vi "oa_Init N Channel Analog Tacho Process Paramters.vi"(6 "slope (Rising)":u16[](array[ring]) items=["Rising", "Falling"], 7 "channel number":i32, 8 "pulse width (2)":i32[](array[numeric]), 9 "pulse/revolution (1)":i32[](array[numeric]), 10 "threshold (auto)":dbl[](array[numeric]) format="%.2f", 11 "missing pulses? (no:F)":bool[](array[boolean])) -> (0 "pulse width out":i32[](array[numeric]), 1 "pulse/revolution out":i32[](array[numeric]), 2 "threshold out":dbl[](array[numeric]) format="%.2f", 3 "missing pulses? out":bool[](array[boolean]), 4 "slope out":u16[](array[ring]) items=["Rising", "Falling"])   [LabVIEW 2017, in "SoundVib_TachProcess.lvlib"]
uses:
  <vilib>/addons/Sound and Vibration/Order Analysis/Tach Process/SoundVib_TachProcess.lvlib
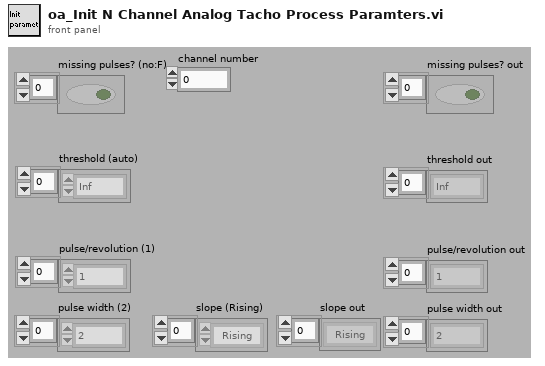
[diagram p1: front panel]
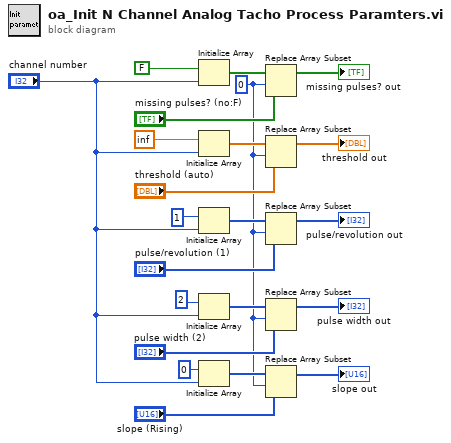
[diagram p0: block diagram]
diagram:
  w4 = 0 ("index")
  n1 = Initialize Array(FALSE, "channel number") -> (w21:bool[])
  n2 = Initialize Array(inf ("element"), "channel number") -> (w17:dbl[])
  n3 = Initialize Array(1, "channel number") -> (w13:i32[])
  n4 = Initialize Array(2, "channel number") -> (w9:i32[])
  n5 = Initialize Array(u16 0 ("element"), "channel number") -> (w5:u16[])
  n6 = Replace Array Subset(array=w21, new element="missing pulses? (no:F)", index=w4) -> (→"missing pulses? out":bool[])
  n7 = Replace Array Subset(array=w17, new element="threshold (auto)", index=w4) -> (→"threshold out":dbl[])
  n8 = Replace Array Subset(array=w13, new element="pulse/revolution (1)", index=w4) -> (→"pulse/revolution out":i32[])
  n9 = Replace Array Subset(array=w9, new element="pulse width (2)", index=w4) -> (→"pulse width out":i32[])
  n10 = Replace Array Subset(array=w5, new element="slope (Rising)", index=w4) -> (→"slope out":u16[])
